vi "Robot Global Data.vi"() -> ()   [LabVIEW 2016]
doc: "This global VI can contain as many global variables as you need. Place a control on the panel, give it a good name. To read or write to it from a VI, drag the icon to the diagram of that VI. You can also drag from the project. Click on the node to change which global you access. You shouldn't have multiple locations writing to a global or it will cause a race-condition."
uses:
  <vilib>/Rock Robotics/WPI/Camera/WPI_CameraImageSize.ctl
  <vilib>/Rock Robotics/WPI/DriverStation/WPI_DriverStationRobotMode2.ctl
panel:
  out "LED Turn On LED":bool
  in  "LED Enum":enum16{""}(ring)
  in  "LED Color":string
  out "LED Black Signal":bool
  out "LED Yellow Signal":bool
  out "LED Purple Signal":bool
  out "LED Blue Signal":bool
  out "LED Green Signal":bool
  out "LED Red Signal":bool
  out "GyroReset":bool
  out "DTRightEncVel":dbl
  out "DTRightEncPos":dbl
  out "DTRightAppliedThrottle":dbl
  out "DTLeftEncVel":dbl
  out "DTLeftEncPos":dbl
  out "DTLeftAppliedThrottle":dbl
  out "xboxBack":bool
  out "ClimberMotorInd":dbl
  in  "ClimberDeployValue":enum16{"Off", "On", "Forward", "Reverse"}(ring)
  out "AutoAngle":dbl
  in  "ClimberMov.AvgLength":dbl
  out "PIDOn":bool
  out "AutoYAxis":dbl
  out "AutoXAxis":dbl
  out "DriveAngle":dbl
  out "GyroYaw(Deg)":dbl
  out "ClimberEncDistance":dbl
  out "ClimberHiSpd":dbl=1.0
  out "ClimberMedSpd":dbl
  out "ClimberLowSpd":dbl
  out "RJYaxis":dbl
  out "RJXaxis":dbl
  out "LJYaxis":dbl
  out "LJXaxis":dbl
  out "xboxRB":bool
  out "xboxLB":bool
  out "xboxY":bool
  out "xboxX":bool
  out "xboxB":bool
  out "xboxA":bool
  out "LJbutton5":bool
  out "LJbutton4":bool
  out "LJbutton3":bool
  out "LJbutton2":bool
  out "LJbutton1":bool
  out "LJbutton0":bool
  out "RJbutton5":bool
  out "RJbutton4":bool
  out "RJbutton3":bool
  out "RJbutton2":bool
  out "RJbutton1":bool
  out "RJbutton0":bool
  in  "Robot Mode":T1
  in  "image size":T2=enum."320x240"
  in  "Enable Vision":bool
  # "LeftJoystick"
  # "RightJoystick"
  # "xboxController"
  # "LED"
  # "Climber"
  # "Gyro Control"
  # "Autonomous"
  # "RobotDrive"
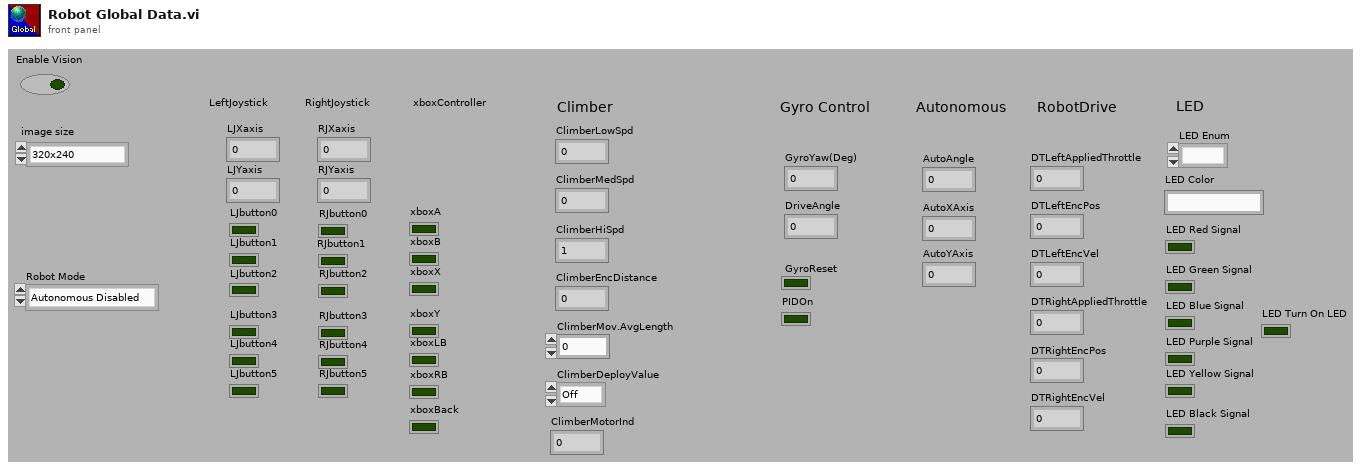
[diagram p1: front panel]
types:
  T1 = typedef "WPI_DriverStationRobotMode2.ctl" = enum16{"Autonomous Disabled", "Autonomous Enabled", "Teleop Disabled", "Teleop Enabled", "Disconnected", "Finish", "Test Disabled", "Test Enabled", "Emergency Stopped"}
  T2 = typedef "WPI_CameraImageSize.ctl" = enum16{"640x480", "320x240", "160x120", "Custom"}
diagram:
